vi "test_deviceManagerMain.vi"(8 "error in (no error)":errorcluster) -> (0 "error out":errorcluster)   [LabVIEW 2020, in "horiba.test.lvlib"]
uses:
  horiba.test.lvlib
  <vilib>/addons/_JKI Toolkits/Caraya/classes/Test/Test.lvclass
panel:
  # "Connector Pane"
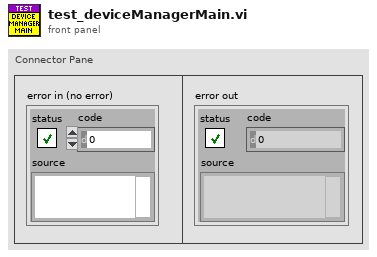
[diagram p1: front panel]
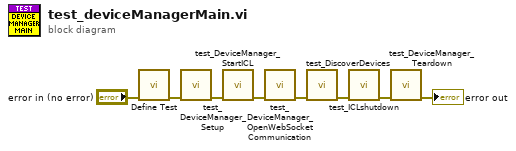
[diagram p0: block diagram]
diagram:
  n1 = call <vilib>:"Define Test.vi"("error in (no error)"="error in (no error)") -> ("error out"=w7:errorcluster)  [unwired: 9 in, 1 out]
  n2 = call "test_DeviceManager_Setup.vi"("error in (no error)"=w7) -> ("error out"=w8:errorcluster)  [unwired: 10 in]
  n3 = call "test_DeviceManager_StartICL.vi"("error in"=w8) -> ("error out"=w1:errorcluster)  [unwired: 10 in]
  n4 = call "test_DeviceManager_OpenWebSocketCommunication.vi"("error in"=w1) -> ("error out"=w6:errorcluster)  [unwired: 10 in]
  n5 = call "test_DiscoverDevices.vi"("error in"=w6) -> ("error out"=w5:errorcluster)  [unwired: 10 in]
  n6 = call "test_ICLshutdown.vi"("error in"=w5) -> ("error out"=w4:errorcluster)  [unwired: 10 in]
  n7 = call "test_DeviceManager_Teardown.vi"("error in"=w4) -> ("error out"=→"error out":errorcluster)  [unwired: 10 in]
